vi "Throw error if MUXed and Connected.vi"(8 "error in (no error)":errorcluster, 9 "Destination":string, 10 "Source":string, 11 "SLSC Switch in":refnum<class "SLSC Switch.lvclass">) -> (0 "error out":errorcluster, 3 "SLSC Switch out":refnum<class "SLSC Switch.lvclass">)   [LabVIEW 2015, in "SLSC Switch.lvlib" / "SLSC Switch.lvclass"]
uses:
  SLSC Switch.lvclass
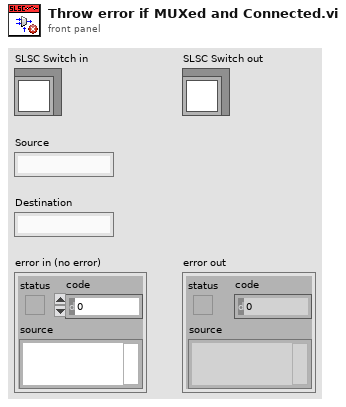
[diagram p1: front panel]
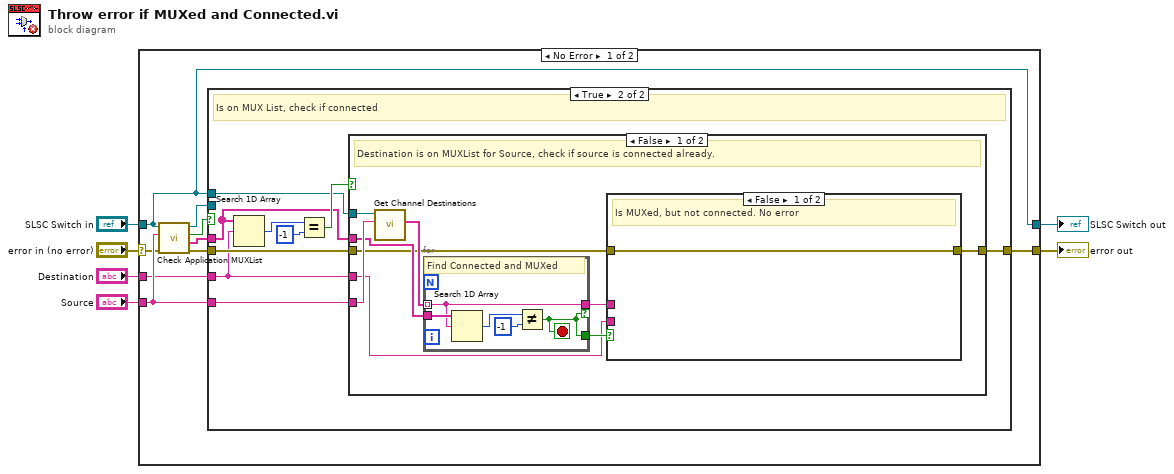
[diagram p0: block diagram]
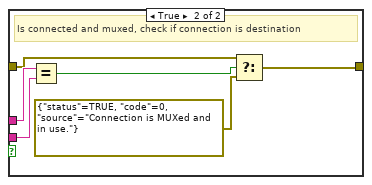
[diagram p3: hidden frame]
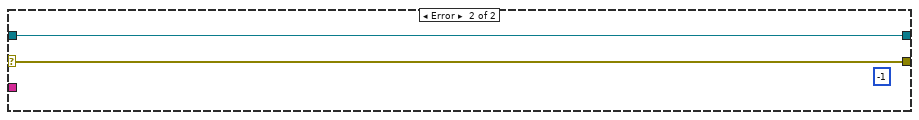
[diagram p5: hidden frame]
diagram:
  n1 = case shown="No Error" "error in (no error)" {
    selector: "error in (no error)" -> [w11 w49]
    tunnel: [w14 w49] -> w5
    tunnel: [w7 w48] -> w3
    tunnel: "SLSC Switch in" -> [w7 w48]
    tunnel: "Source" -> [w15 _]
    tunnel: "Destination" -> [w9 _]
    frame No Error {
      n2 = call "Check Application MUXList.vi"("error in (no error)"=w11, "Source"=w15, "SLSC Switch in"=w7) -> ("error out"=w10:errorcluster, "Destinations"=w8:string[], "found?"=w12:bool, "SLSC Switch out"=w13:refnum<class "SLSC Switch.lvclass">)  [unwired: 4 in, 1 out]
      n3 = case shown="True" w12 {
        tunnel: w13 -> [_ _]
        tunnel: w15 -> [_ w19]
        tunnel: [w16 w22] -> w14
        tunnel: w10 -> [w16 w21]
        tunnel: w9 -> [_ w17]
        tunnel: w8 -> [_ w18]
        tunnel: w7 -> [_ w20]
        frame False {
          # "Is NOT on MUX list, connections are allowed"
        }
        frame True {
          # "Is on MUX List, check if connected"
          n4 = Search 1D Array(1D array=w18, element=w17) -> (index of element=w25:i32)  [unwired: 1 in]
          n5 = Equal?(x=w25, y=-1) -> (x = y?=w23:bool)
          n6 = case shown="False" w23 {
            tunnel: [w26 w47] -> w22
            tunnel: w21 -> [w27 w47]
            tunnel: w20 -> [w34 _]
            tunnel: w19 -> [w33 _]
            tunnel: w18 -> [w31 _]
            tunnel: w17 -> [w28 _]
            frame False {
              # "Destination is on MUXList for Source, check if source is connected already."
              n7 = call "Get Channel Destinations.vi"("Source"=w33, "SLSC Switch in"=w34) -> ("Array"=w32:string[])  [unwired: 9 in]
              n8 = for {
                tunnel: w32 -> [w43] mode=indexing
                tunnel: w31 -> [w46]
                tunnel: [w43] -> w29 if=w42
                tunnel: [w42] -> w30
                stop <- w42 stop-if-true
                # "Find Connected and MUXed"
                n9 = Search 1D Array(1D array=w46, element=w43) -> (index of element=w45:i32)  [unwired: 1 in]
                n10 = Not Equal?(x=w45, y=-1) -> (x != y?=w42:bool)
              }
              n11 = case shown="False" w30 {
                tunnel: w29 -> [_ w41]
                tunnel: w28 -> [_ w40]
                tunnel: w27 -> [w35 w38]
                tunnel: [w35 w36] -> w26
                frame False {
                  # "Is MUXed, but not connected. No error"
                }
                frame True {
                  # "Is connected and muxed, check if connection is destination"
                  n12 = Equal?(x=w41, y=w40) -> (x = y?=w39:bool)
                  n13 = Select(t=w38, s=w39, f=errorcluster {"status"=TRUE, "code"=0, "source"="Connection is MUXed and in use."}) -> (s? t:f=w36:errorcluster)
                }
              }
            }
            frame True {
              # "Destination not on MUXList for Source, no error"
            }
          }
        }
      }
    }
    frame Error {
      (unwired) -1 ("index of element")
    }
  }
  "error out" <- w5
  "SLSC Switch out" <- w3
